vi "Actor Core.vi"(8 "error in":errorcluster, 11 "Nested in":refnum<class "GUI SeñalActualizable.lvclass">) -> (0 "error out":errorcluster, 3 "Actor out":refnum<class "Actor.lvclass">)   [LabVIEW 2020, in "GUI SeñalActualizable.lvlib" / "GUI SeñalActualizable.lvclass"]
doc: "(<B>Filename</B>: Actor Framework.lvlib:Actor.lvclass:Actor Core.vi)\n\nReceives messages to the actor, reacts to them, and initiates any error handling that may shut the actor down.\n\nDescendant classes may override this VI to append parallel tasks for the actor to complete while it handles messages. Overrides use the Call Parent Method node."
uses:
  C:/Program Files (x86)/National Instruments/LabVIEW 2020/vi.lib/ActorFramework/Actor/Actor.lvclass
  <vilib>/ActorFramework/Actor/Actor.lvclass
  Guardar TextoPlano/Guardar TextoPlano/Guardar TextoPlano.lvclass
  Guardar Tipo CSV/Guardar Tipo CSV/Guardar Tipo CSV.lvclass
  <vilib>/ActorFramework/Actor/Actor.lvclass/Actor.ctl
  <vilib>/ActorFramework/Message Enqueuer/Message Enqueuer.lvclass/Message Enqueuer.ctl
  Guardar TextoPlano/Guardar TextoPlano Messages/Enviar Iniciar Guardado Msg/Enviar Iniciar Guardado Msg.lvclass/Enviar Iniciar Guardado Msg.ctl
  Guardar TextoPlano/Guardar TextoPlano Messages/DataAndSave Msg/DataAndSave Msg.lvclass/DataAndSave Msg.ctl
  Guardar Tipo CSV/Guardar Tipo CSV Messages/Start Save Msg/Start Save Msg.lvclass/Start Save Msg.ctl
  Guardar Tipo CSV/Guardar Tipo CSV Messages/Enviar datos Msg/Enviar datos Msg.lvclass/Enviar datos Msg.ctl
  <vilib>/ActorFramework/Message Enqueuer/Init from Existing Queue.vi
  <vilib>/ActorFramework/Message Enqueuer/Enqueue.vi
  <vilib>/ActorFramework/Stop Msg/Stop Msg.lvclass
  C:/Program Files (x86)/National Instruments/LabVIEW 2020/vi.lib/ActorFramework/Message/Message.lvclass
  Guardar TextoPlano/Guardar TextoPlano Messages/Enviar Iniciar Guardado Msg/Enviar Iniciar Guardado Msg.lvclass
  Guardar TextoPlano/Guardar TextoPlano Messages/DataAndSave Msg/DataAndSave Msg.lvclass
  Guardar Tipo CSV/Guardar Tipo CSV Messages/Start Save Msg/Start Save Msg.lvclass
  Guardar Tipo CSV/Guardar Tipo CSV Messages/Enviar datos Msg/Enviar datos Msg.lvclass
  <vilib>/ActorFramework/Message Priority Queue/Priority Enqueue.vi
  <vilib>/ActorFramework/Message Enqueuer/Message Enqueuer.lvclass
panel:
  in  "Parametros":T1
  in  "Save Button":bool
  in  "Tipo de archivo":enum16{"Txt", "CSV"}(ring)
  in  "Path":path
  in  "Exit":bool
  in  "Stop":bool
  in  "Start":bool
  out "Waveform Graph":waveform(dbl)(graph)
  # "Grafica de Funciones"
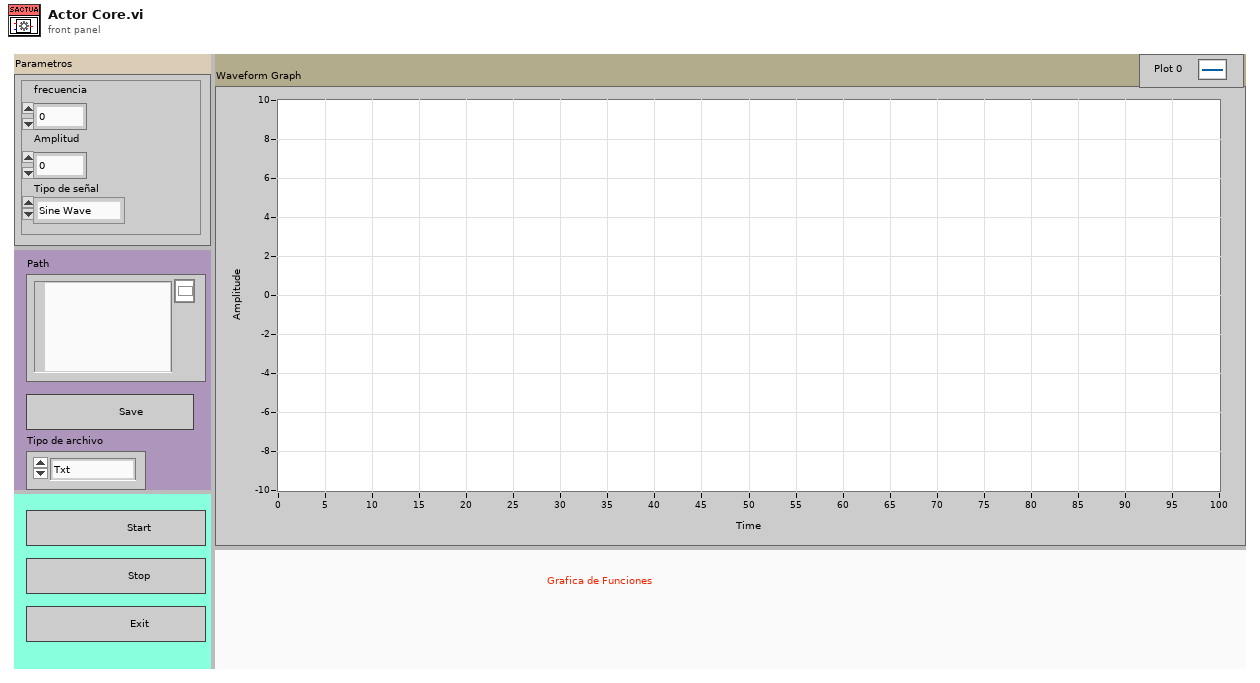
[diagram p1: front panel]
types:
  T1 = cluster{"frecuencia":dbl, "Amplitud":dbl, "Tipo de señal":enum16{"Sine Wave", "Triangle Wave", "Square Wave", "Sawtooth Wave"}}
  T2 = cluster{"Stop":refnum<user-event>, "Waveform Grafica":refnum<user-event>}
  T3 = enum16{"Sine Wave", "Triangle Wave", "Square Wave", "Sawtooth Wave"}
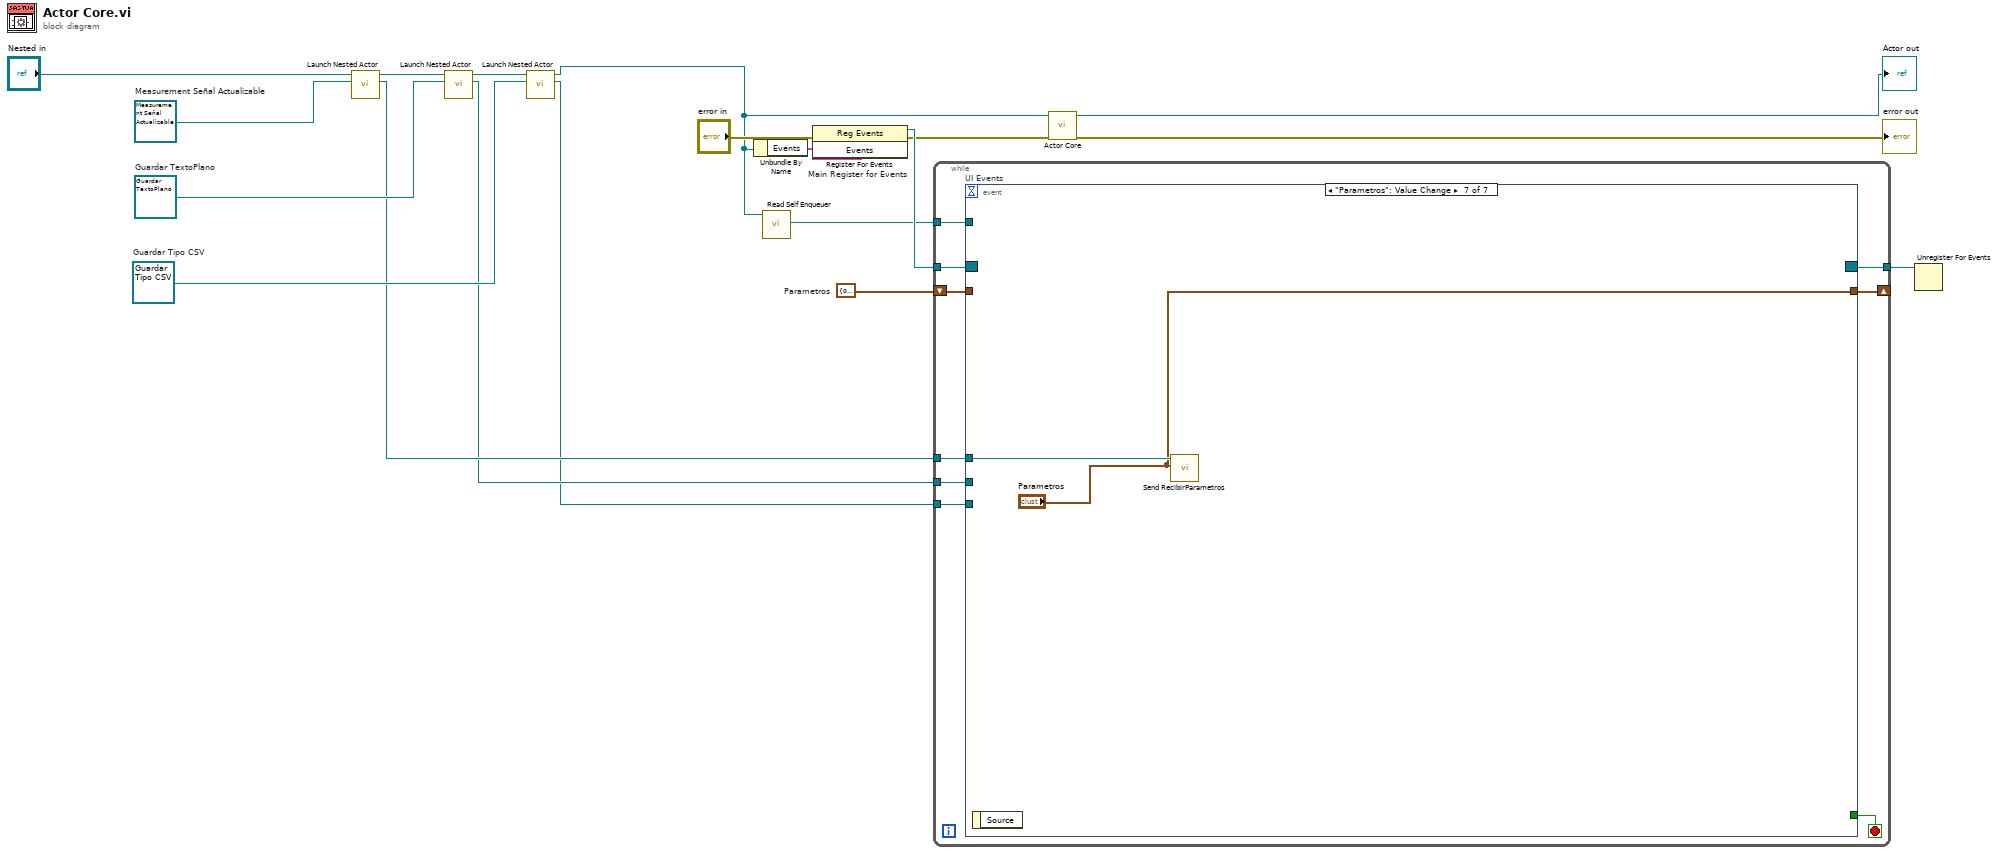
[diagram p0: block diagram]
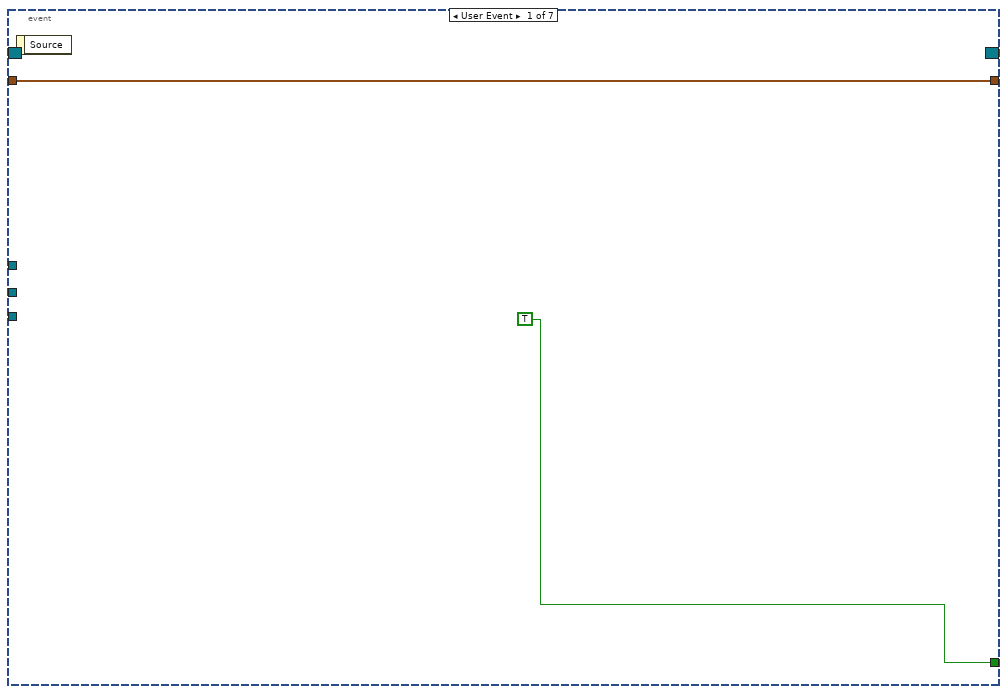
[diagram p2: hidden frame]
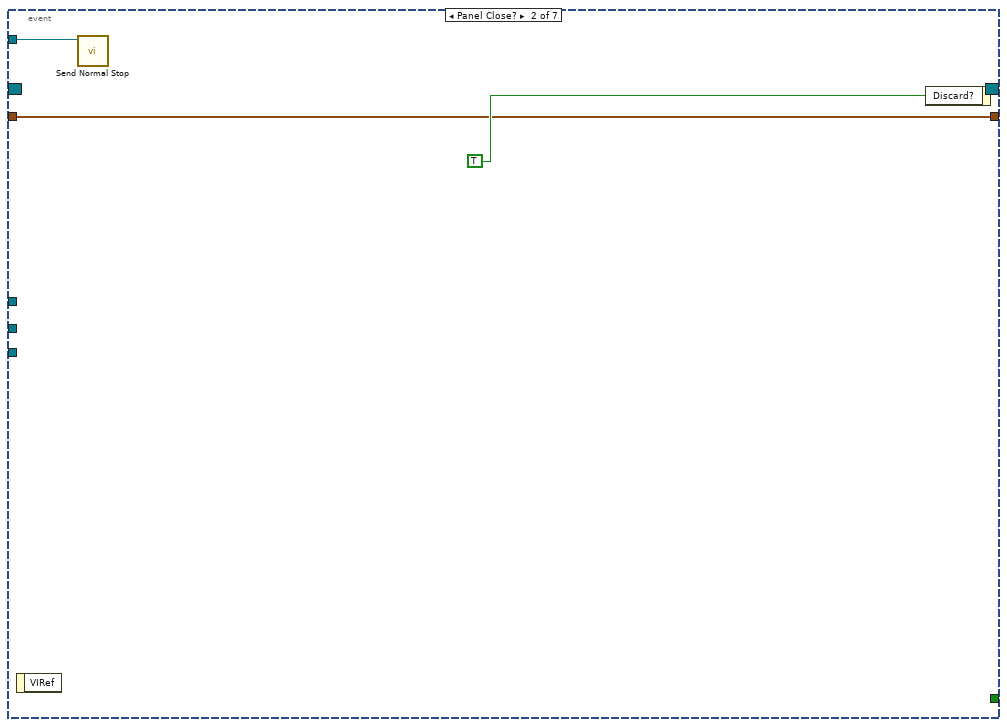
[diagram p3: hidden frame]
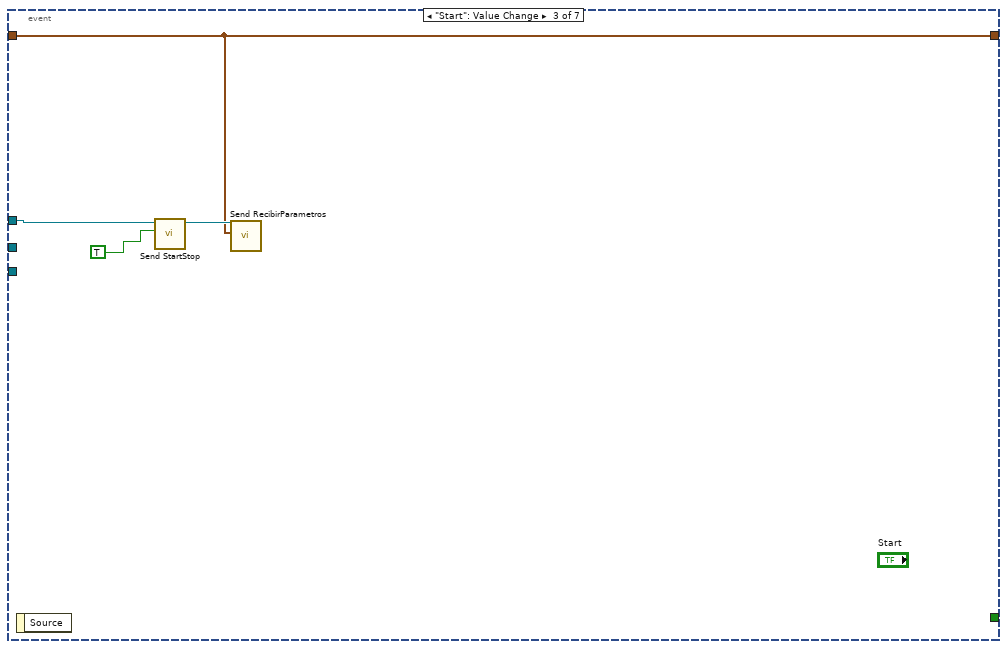
[diagram p4: hidden frame]
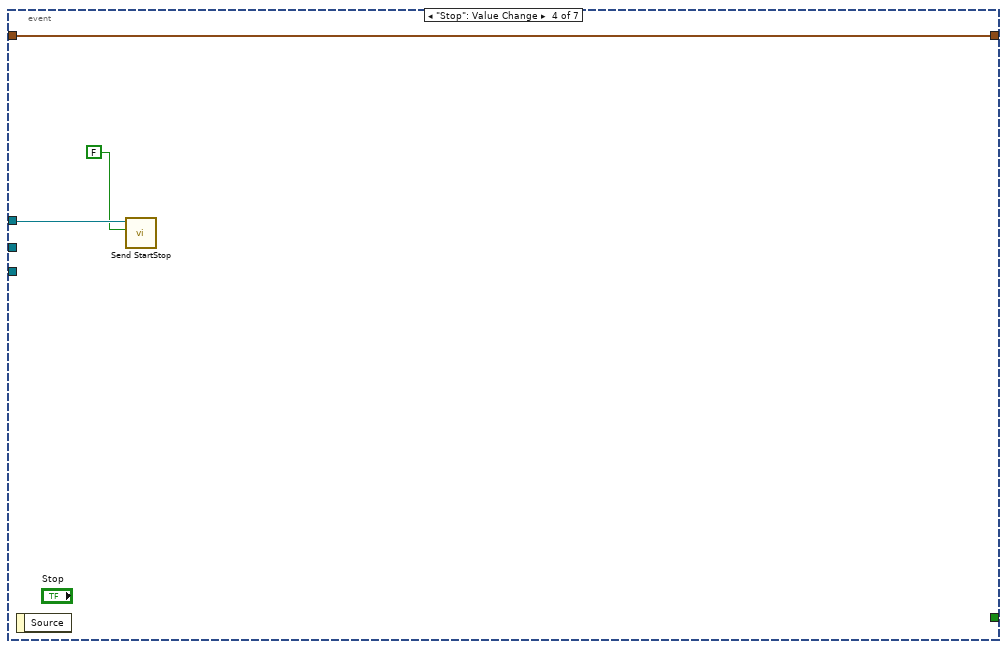
[diagram p5: hidden frame]
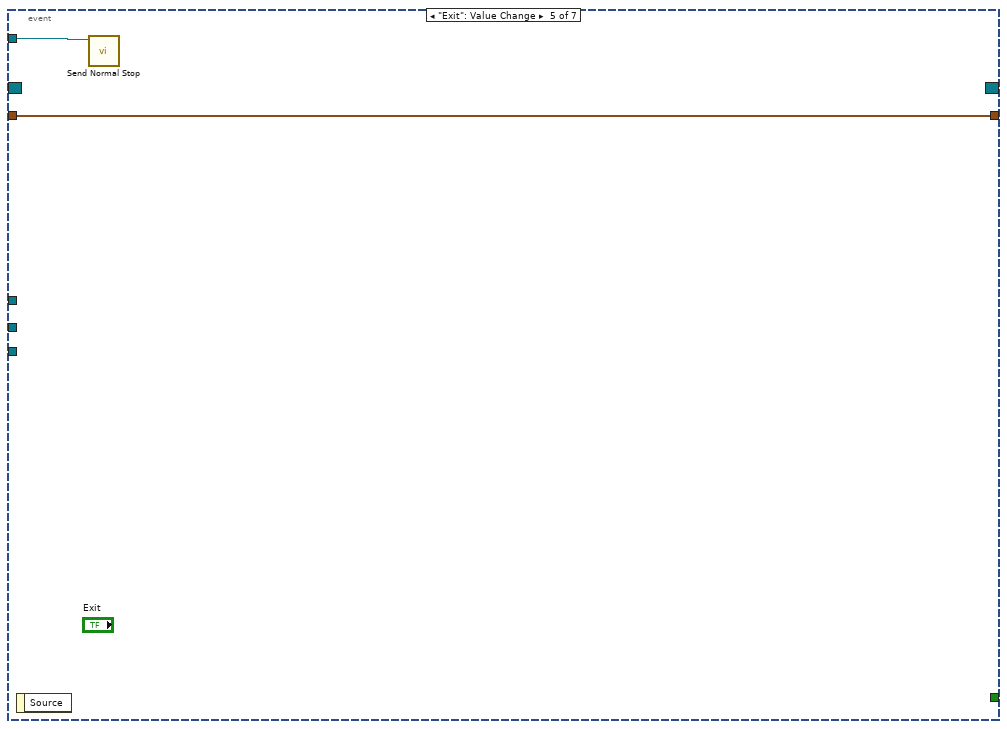
[diagram p6: hidden frame]
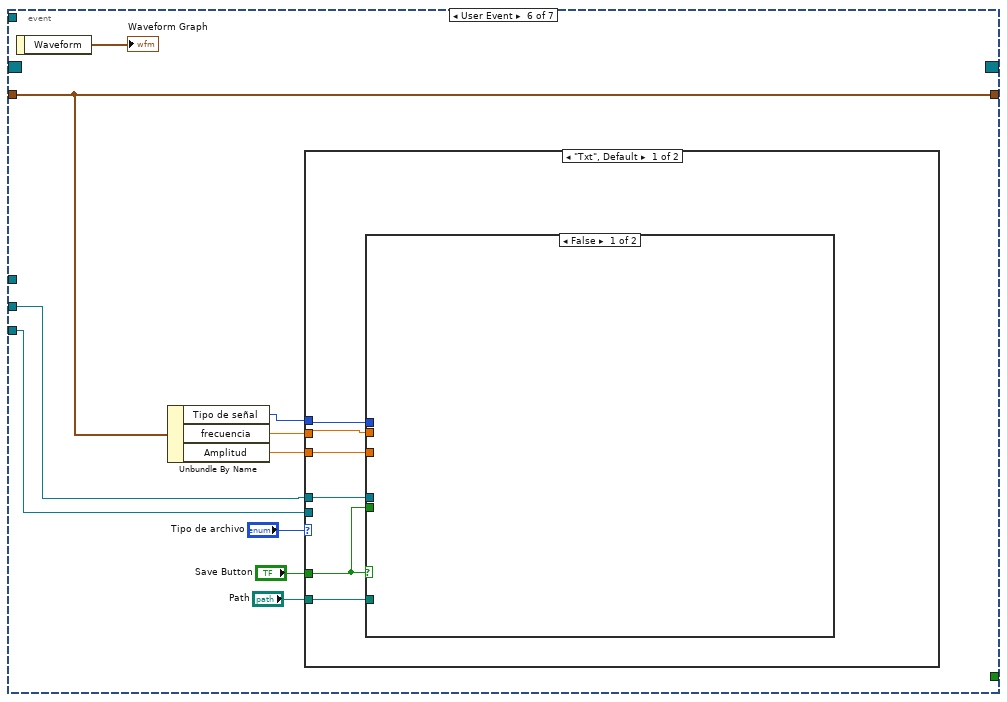
[diagram p7: hidden frame]
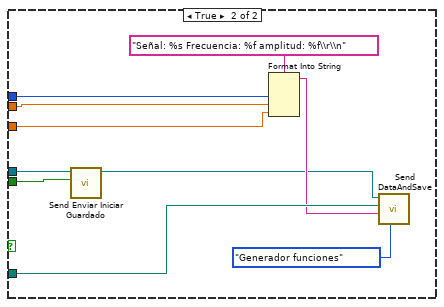
[diagram p8: hidden frame]
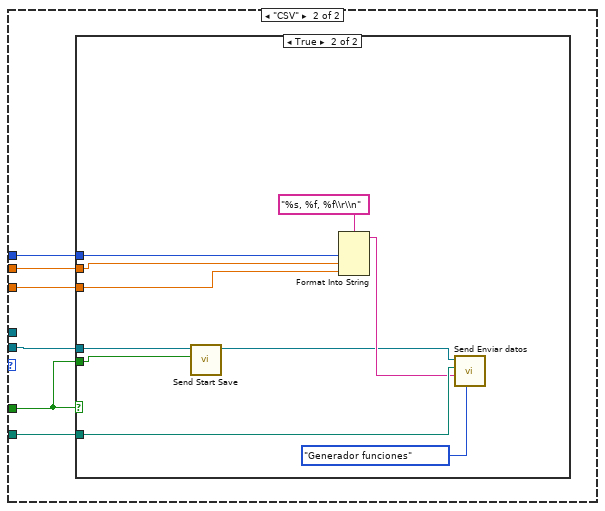
[diagram p9: hidden frame]
diagram:
  w6 = T1 {"frecuencia"=0.0, "Amplitud"=0.0, "Tipo de señal"=enum."Sine Wave"}  # Parametros
  w11 = refnum<class "Measurement Señal Actualizable.lvclass"> refnum  # Measurement Señal Actualizable
  w7 = refnum<class "Guardar Tipo CSV.lvclass"> refnum  # Guardar Tipo CSV
  w8 = refnum<class "Guardar TextoPlano.lvclass"> refnum  # Guardar TextoPlano
  n1 = call <vilib>:"Launch Nested Actor.vi"("Nested Actor"=w11, "Caller Actor in"="Nested in") -> ("Nested Actor's Enqueuer"=w5:refnum<class "Message Enqueuer.lvclass">, "Caller Actor out"=w10:refnum<class "GUI SeñalActualizable.lvclass">)  [unwired: 7 in, 1 out]
  n2 = call <vilib>:"Launch Nested Actor.vi"("Nested Actor"=w8, "Caller Actor in"=w10) -> ("Nested Actor's Enqueuer"=w4:refnum<class "Message Enqueuer.lvclass">, "Caller Actor out"=w9:refnum<class "GUI SeñalActualizable.lvclass">)  [unwired: 7 in, 1 out]
  n3 = call <vilib>:"Launch Nested Actor.vi"("Nested Actor"=w7, "Caller Actor in"=w9) -> ("Nested Actor's Enqueuer"=w3:refnum<class "Message Enqueuer.lvclass">, "Caller Actor out"=w2:refnum<class "GUI SeñalActualizable.lvclass">)  [unwired: 7 in, 1 out]
  n4 = Unbundle By Name(w2) -> ("Events"=w1:T2)
  n5 = call <vilib>:"Read Self Enqueuer.vi"("Actor"=w2) -> ("Self Enqueuer"=w15:refnum<class "Message Enqueuer.lvclass">)  [unwired: 10 in]
  n6 = register-events "Main Register for Events"(error in="error in", w1) -> (reference out=w17:refnum<event-registration>, error out=w13:errorcluster)  [unwired: 1 in]
  n7 = while {
    tunnel: w17 -> [w28]
    tunnel: [w26] -> w16
    tunnel: w15 -> [w25]
    shift-right: [w23] -> _
    shift-left: w6 -> [w24]
    tunnel: w5 -> [w22]
    tunnel: w4 -> [w21]
    tunnel: w3 -> [w20]
    stop <- w27 stop-if-true
    n8 = event "UI Events" shown="[6] \"Parametros\": Value Change" {
      selector: w28 -> [_ _ _ _ _ _ _]
      dyn-events: [_ _ _ _ _ _ _] -> w26
      timeout: _ -> [_ _ _ _ _ _ _]
      tunnel: [TRUE _ _ _ _ _ _] -> w27
      tunnel: w25 -> [_ w32 _ _ w42 _ _]
      tunnel: w24 -> [w29 w31 w35 w38 w41 w51 _]
      tunnel: [w29 w31 w35 w38 w41 w51 "Parametros"] -> w23
      tunnel: w22 -> [_ _ w34 w40 _ _ w86]
      tunnel: w21 -> [_ _ _ _ _ w47 _]
      tunnel: w20 -> [_ _ _ _ _ w48 _]
      event User Event {
        n9 = event-data() -> ()  [unwired: 1 in, 1 out]
      }
      event Panel Close? {
        n10 = event-data() -> ()  [unwired: 1 in, 1 out]
        n11 = call <vilib>:"Send Normal Stop.vi"("Message Enqueuer"=w32) -> ()  [unwired: 10 in, 1 out]
        n12 = event-data("Discard?"=TRUE) -> ()  [unwired: 1 in, 1 out]
      }
      event "Start": Value Change {
        n13 = event-data() -> ()  [unwired: 1 in, 1 out]
        n14 = call "Send StartStop.vi"("Start/Stop"=TRUE, "Message Enqueuer"=w34) -> ("Message Enqueuer out"=w36:refnum<class "Message Enqueuer.lvclass">)  [unwired: 8 in, 1 out]
        n15 = call "Send RecibirParametros.vi"("Parametros"=w35, "Message Enqueuer"=w36) -> ()  [unwired: 8 in, 2 out]
      }
      event "Stop": Value Change {
        n16 = event-data() -> ()  [unwired: 1 in, 1 out]
        n17 = call "Send StartStop.vi"("Start/Stop"=FALSE, "Message Enqueuer"=w40) -> ()  [unwired: 8 in, 2 out]
      }
      event "Exit": Value Change {
        n18 = event-data() -> ()  [unwired: 1 in, 1 out]
        n19 = call <vilib>:"Send Normal Stop.vi"("Message Enqueuer"=w42) -> ()  [unwired: 10 in, 1 out]
      }
      event User Event {
        n20 = event-data() -> ("Waveform"=→"Waveform Graph":waveform(dbl))  [unwired: 1 in]
        n21 = Unbundle By Name(w51) -> ("Tipo de señal"=w45:T3, "frecuencia"=w44:dbl, "Amplitud"=w43:dbl)
        n22 = case shown="\"Txt\", Default" "Tipo de archivo" {
          tunnel: "Save Button" -> [w57 w73]
          tunnel: w48 -> [_ w74]
          tunnel: w47 -> [w58 _]
          tunnel: "Path" -> [w56 w72]
          tunnel: w45 -> [w55 w71]
          tunnel: w44 -> [w54 w70]
          tunnel: w43 -> [w53 w69]
          frame "Txt", Default {
            n23 = case shown="False" w57 {
              tunnel: w58 -> [_ w68]
              tunnel: w57 -> [_ w67]
              tunnel: w56 -> [_ w65]
              tunnel: w55 -> [_ w64]
              tunnel: w54 -> [_ w63]
              tunnel: w53 -> [_ w62]
              frame False {
              }
              frame True {
                n24 = call "Send Enviar Iniciar Guardado.vi"("Save?"=w67, "Message Enqueuer"=w68) -> ("Message Enqueuer out"=w59:refnum<class "Message Enqueuer.lvclass">)  [unwired: 8 in, 1 out]
                n25 = Format Into String(format string="Señal: %s Frecuencia: %f amplitud: %f\\r\\n", w64, w63, w62) -> (resulting string=w60:string)  [unwired: 2 in, 1 out]
                n26 = call "Send DataAndSave.vi"("Proviene de?"=enum16{"Contador", "Generador funciones"}."Generador funciones", "Dato"=w60, "Path"=w65, "Message Enqueuer"=w59) -> ()  [unwired: 6 in, 2 out]
              }
            }
          }
          frame "CSV" {
            n27 = case shown="True" w73 {
              tunnel: w74 -> [_ w84]
              tunnel: w73 -> [_ w83]
              tunnel: w72 -> [_ w82]
              tunnel: w71 -> [_ w81]
              tunnel: w70 -> [_ w80]
              tunnel: w69 -> [_ w79]
              frame False {
              }
              frame True {
                n28 = call "Send Start Save.vi"("Save?"=w83, "Message Enqueuer"=w84) -> ("Message Enqueuer out"=w75:refnum<class "Message Enqueuer.lvclass">)  [unwired: 8 in, 1 out]
                n29 = Format Into String(format string="%s, %f, %f\\r\\n", w81, w80, w79) -> (resulting string=w76:string)  [unwired: 2 in, 1 out]
                n30 = call "Send Enviar datos.vi"("Proviene de?"=enum16{"Contador", "Generador funciones"}."Generador funciones", "Dato"=w76, "Path"=w82, "Message Enqueuer"=w75) -> ()  [unwired: 6 in, 2 out]
              }
            }
          }
        }
      }
      event "Parametros": Value Change {
        n31 = event-data() -> ()  [unwired: 1 in, 1 out]
        n32 = call "Send RecibirParametros.vi"("Parametros"="Parametros", "Message Enqueuer"=w86) -> ()  [unwired: 8 in, 2 out]
      }
    }
  }
  n33 = call-parent "Actor Core.vi"("error in"=w13, "Actor in"=w2) -> ("error out"=→"error out":errorcluster, "Actor out"=→"Actor out":refnum<class "Actor.lvclass">)  [unwired: 8 in]
  n34 = Unregister For Events(event registration refnum=w16) -> ()  [unwired: 1 in, 1 out]
